vi "反转判断1.vi"(6 "重置？":bool, 8 "error in (no error)":errorcluster caption="错误输入（无错误）", 9 "反转判断条件1":T1, 10 "传感器数据":dbl[](array[numeric]), 11 "Message Queues":T2 caption="消息队列") -> (0 "error out":errorcluster caption="错误输出", 2 "反转":bool)   [LabVIEW 2015, in "Action.lvlib"]
uses:
  Action.lvlib
  support/Message Queue/All Message Queues.ctl
  support/Message Queue/Message Cluster.ctl
  support/Message Queue/Enqueue Message (Single).vi
  support/Message Queue/Message Queue.lvlib
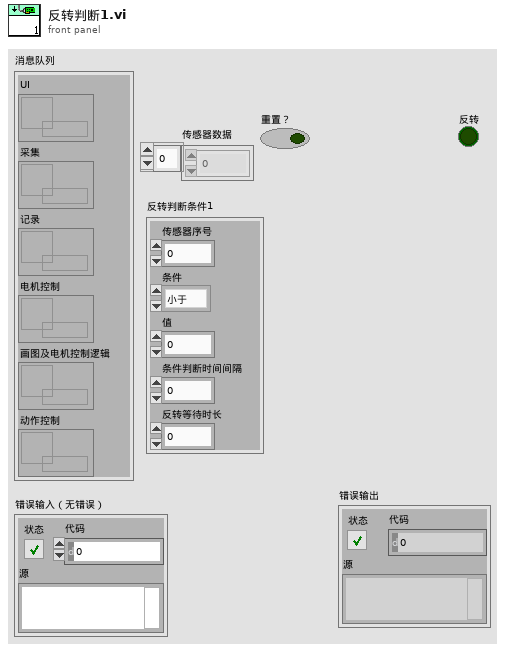
[diagram p1: front panel]
types:
  T1 = typedef "Action.lvlib/反转判断条件1.ctl" = cluster{"传感器序号":i32, "条件":enum16{"小于", "大于", "等于"}, "值":dbl, "条件判断时间间隔":i32, "反转等待时长":i32}
  T2 = typedef "Message Queue.lvlib/All Message Queues.ctl" = cluster{"UI":refnum<queue>, "Acquisition":refnum<queue>, "Logging":refnum<queue>, "MotorCtrl":refnum<queue>, "plot logic":refnum<queue>, "Action Control":refnum<queue>}
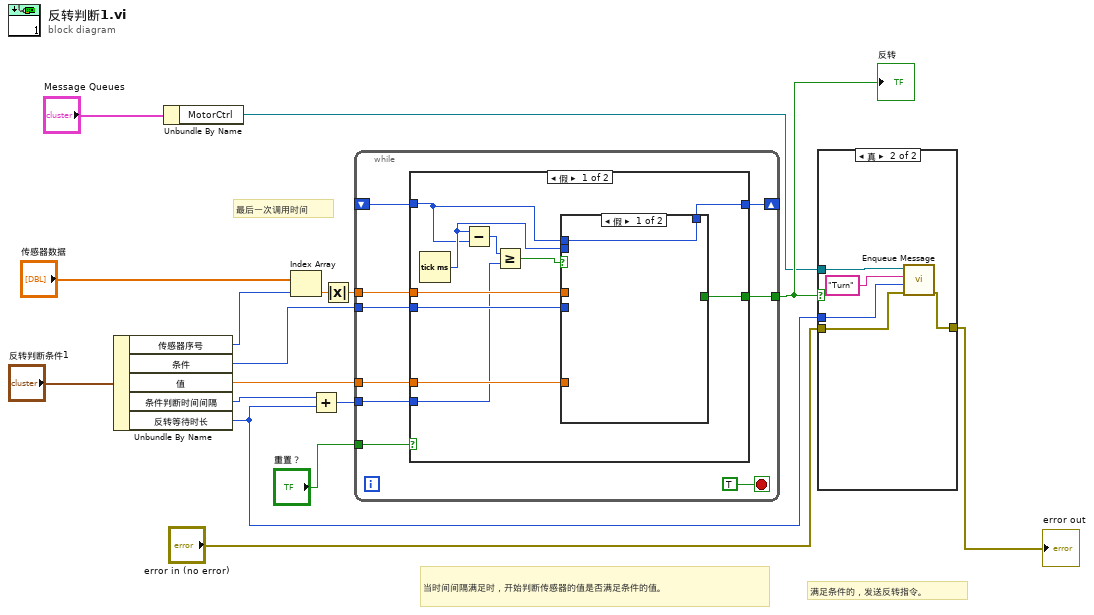
[diagram p0: block diagram]
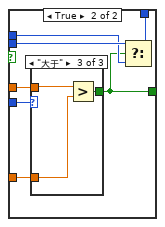
[diagram p3: hidden frame]
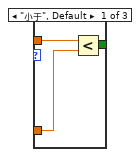
[diagram p4: hidden frame]
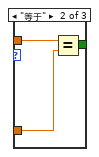
[diagram p5: hidden frame]
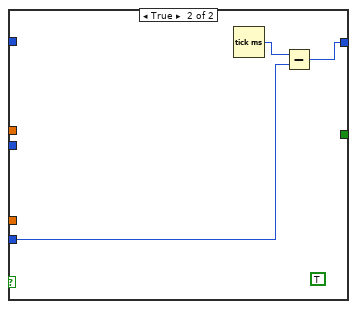
[diagram p6: hidden frame]
diagram:
  # "满足条件的，发送反转指令。"
  # "当时间间隔满足时，开始判断传感器的值是否满足条件的值。"
  # "最后一次调用时间"
  n1 = Unbundle By Name("反转判断条件1") -> ("传感器序号"=w13:i32, "条件"=w12:enum16{"小于", "大于", "等于"}, "值"=w11:dbl, "条件判断时间间隔"=w3:i32, "反转等待时长"=w2:i32)
  n2 = Unbundle By Name("Message Queues") -> ("MotorCtrl"=w9:refnum<queue>)
  n3 = Index Array(array="传感器数据", index=w13) -> (element=w6:dbl)
  n4 = Add(x=w3, y=w2) -> (x+y=w4:i32)
  n5 = Absolute Value(x=w6) -> (abs(x)=w5:dbl)
  n6 = while {
    tunnel: w12 -> [w25]
    tunnel: w5 -> [w24]
    tunnel: w11 -> [w23]
    shift-right: [w22] -> _
    shift-left: _ -> [w21]
    tunnel: w4 -> [w20]
    tunnel: [w19] -> w10
    tunnel: "重置？" -> [w17]
    stop <- TRUE stop-if-true
    n7 = case shown="假" w17 {
      tunnel: w25 -> [w35 _]
      tunnel: w24 -> [w34 _]
      tunnel: w23 -> [w33 _]
      tunnel: [w28 w53] -> w22
      tunnel: w21 -> [w29 _]
      tunnel: w20 -> [w27 w54]
      tunnel: [w31 _] -> w19
      frame False {
        n8 = Tick Count (ms)() -> (millisecond timer value=w30:u32)
        n9 = Subtract(x=w30, y=w29) -> (x-y=w32:u32)
        n10 = Greater Or Equal?(x=w32, y=w27) -> (x >= y?=w26:bool)
        n11 = case shown="假" w26 {
          tunnel: w35 -> [_ w43]
          tunnel: w34 -> [_ w42]
          tunnel: w33 -> [_ w41]
          tunnel: [_ w37] -> w31
          tunnel: w30 -> [_ w40]
          tunnel: w29 -> [w36 w39]
          tunnel: [w36 w38] -> w28
          frame False {
          }
          frame True {
            n12 = case shown="\"大于\"" w43 {
              tunnel: w42 -> [w46 w49 w52]
              tunnel: w41 -> [w45 w48 w51]
              tunnel: [w44 w47 w50] -> w37
              frame "小于", Default {
                n13 = Less?(x=w46, y=w45) -> (x < y?=w44:bool)
              }
              frame "等于" {
                n14 = Equal?(x=w49, y=w48) -> (x = y?=w47:bool)
              }
              frame "大于" {
                n15 = Greater?(x=w52, y=w51) -> (0:w50:bool)
              }
            }
            n16 = Select(t=w40, s=w37, f=w39) -> (s? t:f=w38:u32)
          }
        }
      }
      frame True {
        (unwired) TRUE
        n17 = Tick Count (ms)() -> (millisecond timer value=w55:u32)
        n18 = Subtract(x=w55, y=w54) -> (x-y=w53:u32)
      }
    }
  }
  "反转" <- w10
  n19 = case shown="真" w10 {
    tunnel: w9 -> [_ w61]
    tunnel: "error in (no error)" -> [w56 w60]
    tunnel: [w56 w59] -> w7
    tunnel: w2 -> [_ w57]
    frame False {
    }
    frame True {
      n20 = call-poly "Enqueue Message.vi"("error in (no error)"=w60, "Message Data"=w57, "Message"="Turn", "Message Queue"=w61) -> ("error out"=w59:errorcluster)  [unwired: 6 in, 1 out]
    }
  }
  "error out" <- w7
